vi "TEST - Cluster to VArray.vi"(8 "error in (no error)":errorcluster) -> (0 "error out":errorcluster, 2 "pass":bool)   [LabVIEW 2020]
uses:
  source/library/oglib_lvdata.lvlib
panel:
  out "Expected Result":i32[](array[numeric])
  out "Result":i32[](array[numeric])
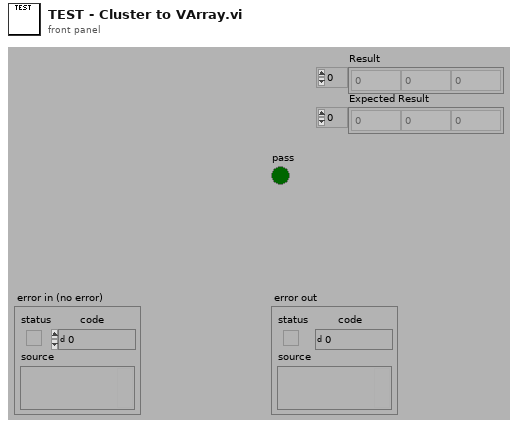
[diagram p1: front panel]
types:
  T1 = cluster{"code 1":i32, "code 2":i32, "code 3":i32}
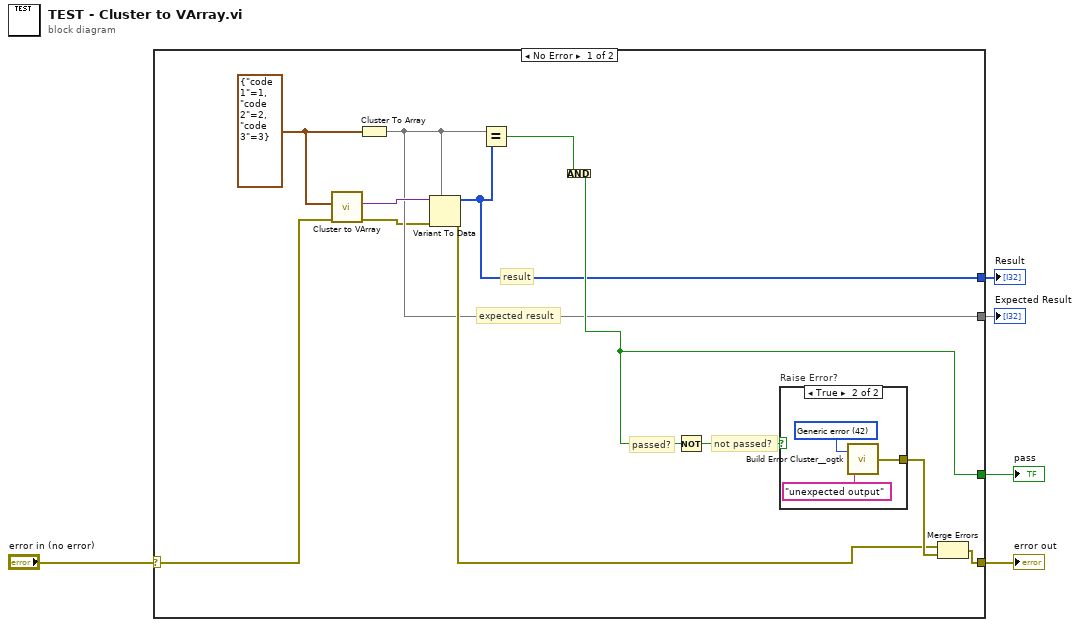
[diagram p0: block diagram]
diagram:
  n1 = case shown="No Error" "error in (no error)" {
    selector: "error in (no error)" -> [w7 w21]
    tunnel: [w14 _] -> w5
    tunnel: [w17 w21] -> w3
    tunnel: [w11 _] -> w2
    tunnel: [w8 _] -> w1
    frame No Error {
      w9 = T1 {"code 1"=1, "code 2"=2, "code 3"=3}
      # "result"
      # "expected result"
      # "not passed?"
      # "passed?"
      n2 = call "Cluster to VArray.vi"("error in (no error)"=w7, "Cluster"=w9) -> ("error out"=w6:errorcluster, "VArray"=w10:variant)  [unwired: 8 in]
      n3 = Cluster To Array(cluster=w9) -> (array=w8:i32[])
      n4 = Variant To Data(error in=w6, type=w8, Variant=w10) -> (data=w11:i32[], error out=w12:errorcluster)
      n5 = Equal?(x=w8, y=w11) -> (x = y?=w13:bool)
      n6 = Compound Arithmetic op=AND(w13) -> (w14:bool)
      n7 = Not(x=w14) -> (.not. x?=w15:bool)
      n8 = case "Raise Error?" shown="True" w15 {
        tunnel: [_ w18] -> w16
        frame False {
        }
        frame True {
          w19 = 42 items=["No error", "Argument error", "Memory is full", "Out of zone", "End of file", "File already open", "Generic file I/O error", "File not found", "File permission error", "Disk is full", "Duplicate path", "Too many files open", "System feature not enabled", "Resource file not found", "Cannot add resource", "Resource not found", "Image not found", "Image memory error", "Pen does not exist", "Config type invalid", "Config token not found", "Config parse error", "Config memory error", "Bad external code format", "Bad external code offset", "External code not present", "Null window", "Destroy window error", "Null menu", "Print aborted", "Bad print record", "Print driver error", "Windows error during printing", "Memory error during printing", "Print dialog error", "Generic print error", "Invalid device refnum", "Device not found", "Device parameter error", "Device unit error", "Cannot open device", "Device call aborted", "Generic error", "Cancelled by user", "Object ID too low", "Object ID too high", "Object not in heap", "Unknown heap", "Unknown object (invalid DefProc)", "Unknown object (DefProc not in table)", "Message out of range", "Invalid (null) method", "Unknown message", "Manager call not supported", "Bad address", "Network operation in progress", "Network operation timed out", "Connection is busy", "Network attribute not supported", "Network error", "Address in use", "System out of memory", "Connection aborted", "Connection refused", "Not connected", "Already connected", "Connection closed", "Initialization error (interapplication manager)", "Bad occurrence", "Wait on unbound occurrence handler", "Occurrence queue overflow", "Datalog type conflict", "Unused", "Unrecognized type (interapplication manager)", "Memory corrupt", "Failed to make temporary DLL", "Old CIN version", "Drag socket not found", "Failed to load drop-object", "Failed to register OLE object", "Failed to release OLE object", "Format specifier type mismatch", "Unknown format specifier", "Too few format specifiers", "Too many format specifiers", "Scan failed", "Newer CIN version", "Error converting to variant", "Runtime menu error", "Password tampered", "Variant attribute not found", "Incompatible variant data type", "Event data is not available", "Event Store is not present", "Occurrence is not found", "Event Queue is not created", "Event info is not available", "Refnum passed is NULL", "Error retrieving Class GUID", "Error retrieving CoClass GUID", "Error retrieving TypeLib GUID.", "Bad built application magic bytes.", "Specific driver is different from the specific driver associated with the Logical Name.", "There is no session opened to the class driver.", "Max Error", "MAX - Error with config objects", "MAX - Error loading configuration", "MAX - Group not supported"]
          n9 = call <userlib>:"Build Error Cluster__ogtk.vi"("String to Prepend to source (\"\")"="unexpected output" ("String to Prepend to source (\"\")"), "code"=w19) -> ("error out"=w18:errorcluster)
        }
      }
      n10 = Merge Errors(w12, w16) -> (w17:errorcluster)
    }
    frame Error {
    }
  }
  "pass" <- w5
  "error out" <- w3
  "Result" <- w2
  "Expected Result" <- w1
